vi "RemoveBadPoints.vi"(9 "limits":T1={"X upper limit"=215.0, "X lower limit"=120.0, "Y upper limit"=35.0, "Y lower limit"=0.0} {"Y lower limit" format="%#_13g"; "Y upper limit" format="%#_13g"; "X lower limit" format="%#_13g"; "X upper limit" format="%#_13g"}, 10 "Y Array":dbl[](array[numeric]), 11 "X Array":dbl[](array[numeric])) -> (2 "Y Array":dbl[](array[numeric]), 3 "X Array":dbl[](array[numeric]))   [LabVIEW 2016]
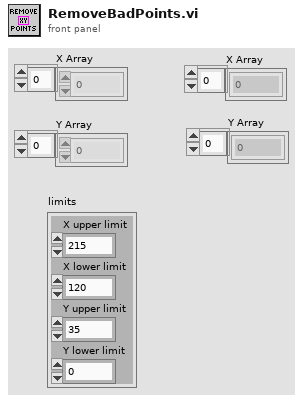
[diagram p1: front panel]
types:
  T1 = cluster{"X upper limit":dbl, "X lower limit":dbl, "Y upper limit":dbl, "Y lower limit":dbl}
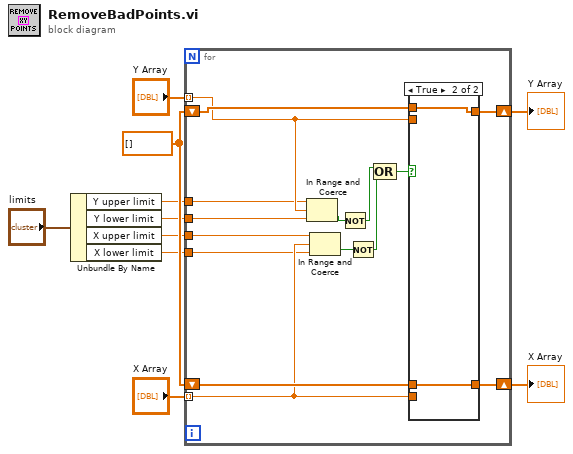
[diagram p0: block diagram]
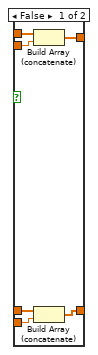
[diagram p2: hidden frame]
diagram:
  w10 = dbl[] []
  n1 = Unbundle By Name("limits") -> ("Y upper limit"=w4:dbl, "Y lower limit"=w3:dbl, "X upper limit"=w2:dbl, "X lower limit"=w1:dbl)
  n2 = for {
    tunnel: "Y Array" -> [w16] mode=indexing
    tunnel: "X Array" -> [w21] mode=indexing
    shift-right: [w24] -> w8
    shift-left: w10 -> [w23]
    shift-right: [w22] -> w9
    shift-left: w10 -> [w25]
    tunnel: w4 -> [w14]
    tunnel: w3 -> [w13]
    tunnel: w2 -> [w12]
    tunnel: w1 -> [w11]
    n3 = In Range and Coerce(upper limit=w14, x=w16, lower limit=w13) -> (In Range?=w17:bool)  [unwired: 1 out]
    n4 = In Range and Coerce(upper limit=w12, x=w21, lower limit=w11) -> (In Range?=w19:bool)  [unwired: 1 out]
    n5 = Not(x=w17) -> (.not. x?=w15:bool)
    n6 = Not(x=w19) -> (.not. x?=w18:bool)
    n7 = Compound Arithmetic op=OR(w15, w18) -> (w20:bool)
    n8 = case shown="True" w20 {
      tunnel: w21 -> [w31 _]
      tunnel: w16 -> [w30 _]
      tunnel: w25 -> [w29 w32]
      tunnel: [w28 w32] -> w22
      tunnel: [w27 w33] -> w24
      tunnel: w23 -> [w26 w33]
      frame False {
        n9 = Build Array (concatenate)(w29, w30) -> (w28:dbl[])
        n10 = Build Array (concatenate)(w26, w31) -> (w27:dbl[])
      }
      frame True {
      }
    }
  }
  "Y Array" <- w9
  "X Array" <- w8
